vi "Actuators Get Position.vi"(0 "Notifier Name":string, 11 "Error In":errorcluster) -> (4 "Notifier Name Out":string, 8 "Position":dbl[](array[numeric]), 10 "Status Bits":u32[](array[numeric]), 13 "Moving":bool[](array[boolean]), 15 "Error Out":errorcluster)   [LabVIEW 2020]
uses:
  Actuators Controls/Actuators Note Type.ctl
  Actuators Controls/Actuators Actions.ctl
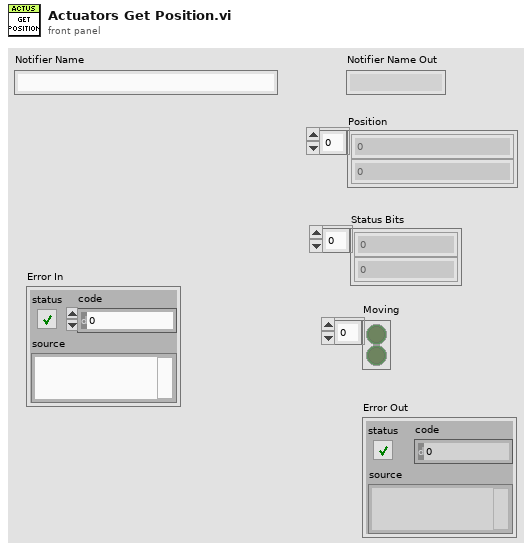
[diagram p1: front panel]
types:
  T1 = typedef "Actuators Note Type.ctl" = cluster{"Actions":T2, "Cmd Received ":bool, "Setpoint":dbl[], "Position":dbl[], "Channel":i32[], "Jog Step":dbl[], "Velocity":dbl[], "Acceleration":dbl[], "Status Bits":u32[], "Moving":bool[]}
  T2 = typedef "Actuators Actions.ctl" = enum16{"Nothing", "Get Position", "Get Acceleration", "Get Velocity", "Get Jog Step", "Set Acceleration", "Set Velocity", "Set Jog Step", "Move Absolute", "Move Relative", "Jog Forward", "Jog Reverse", "Set Moving", "Halt", "Quit"}
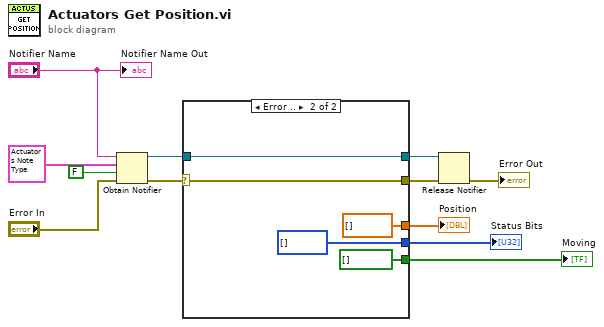
[diagram p0: block diagram]
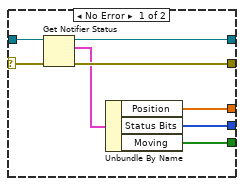
[diagram p2: hidden frame]
diagram:
  n1 = Obtain Notifier(name (unnamed)="Notifier Name", notification data type=T1 {"Actions"=enum."Nothing", "Cmd Received "=FALSE, "Setpoint"=[], "Position"=[], "Channel"=[], "Jog Step"=[], "Velocity"=[], "Acceleration"=[], "Status Bits"=[], "Moving"=[]} ("Actuators Note"), create if not found? (T)=FALSE, error in (no error)="Error In") -> (notifier out=w8:refnum<notifier>, error out=w11:errorcluster)  [unwired: 1 out]
  n2 = case shown="Error .." w11 {
    selector: w11 -> [w19 w24]
    tunnel: w8 -> [w20 w25]
    tunnel: [w18 w25] -> w7
    tunnel: [w17 w24] -> w6
    tunnel: [w15 dbl[] [] ("Position")] -> w4
    tunnel: [w14 u32[] [] ("Status Bits")] -> w2
    tunnel: [w13 bool[] [] ("Moving")] -> w1
    frame No Error {
      n3 = Get Notifier Status(notifier=w20, error in (no error)=w19) -> (notifier out=w18:refnum<notifier>, current notification=w16:T1, error out=w17:errorcluster)  [unwired: 2 out]
      n4 = Unbundle By Name(w16) -> ("Position"=w15:dbl[], "Status Bits"=w14:u32[], "Moving"=w13:bool[])
    }
    frame Error {
    }
  }
  "Position" <- w4
  "Status Bits" <- w2
  "Moving" <- w1
  n5 = Release Notifier(notifier=w7, error in (no error)=w6) -> (error out=→"Error Out":errorcluster)  [unwired: 1 in, 2 out]
  "Notifier Name Out" <- "Notifier Name"
